vi "Set Pump Power.vi"(7 "timeout":i32=1000, 8 "error in":errorcluster, 9 "Power %":dbl=0.15 min=0.15 max=100.0 step=5.0 format="%#_2f", 11 "CAN Session In":T1) -> (0 "error out":errorcluster, 3 "CAN Session Out":T1)   [LabVIEW 2016]
uses:
  Program Files (x86)/National Instruments/LabVIEW 2016/examples/robotics/EPOS2 CANOpen Driver/Low Level VIs/Typedefs/CAN Refnum.ctl
  Program Files (x86)/National Instruments/LabVIEW 2016/examples/robotics/EPOS2 CANOpen Driver/Low Level VIs/Typedefs/CAN Session Pointer.ctl
  Program Files (x86)/National Instruments/LabVIEW 2016/examples/robotics/EPOS2 CANOpen Driver/Low Level VIs/Typedefs/CAN Communication References.ctl
  Program Files (x86)/National Instruments/LabVIEW 2016/examples/robotics/EPOS2 CANOpen Driver/Low Level VIs/Typedefs/kill process notifier array.ctl
  Program Files (x86)/National Instruments/LabVIEW 2016/examples/robotics/EPOS2 CANOpen Driver/Low Level VIs/Typedefs/Write Queue.ctl
  Program Files (x86)/National Instruments/LabVIEW 2016/examples/robotics/EPOS2 CANOpen Driver/Low Level VIs/Typedefs/FPGA CAN Frame Cluster.ctl
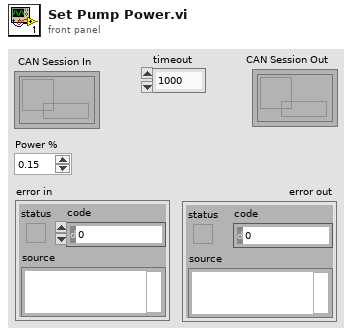
[diagram p1: front panel]
types:
  T1 = typedef "CAN Refnum.ctl" = refnum<k1>
  T2 = typedef "FPGA CAN Frame Cluster.ctl" = cluster{"Timestamp":u64, "Identifier":u32, "Type":u8, "InfoA":u8, "InfoB":u8, "DataLength":u8, "Data":u8[]}
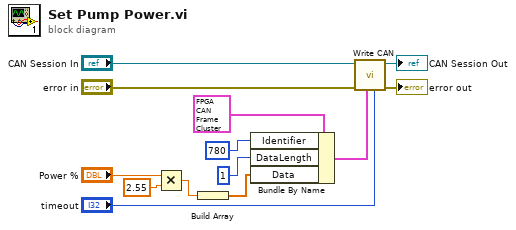
[diagram p0: block diagram]
diagram:
  n1 = Multiply(x="Power %", y=2.55) -> (x*y=w2:dbl)
  n2 = Build Array(w2) -> (w10:dbl[])
  n3 = Bundle By Name(cluster=T2 {"Timestamp"=0, "Identifier"=0, "Type"=0, "InfoA"=0, "InfoB"=0, "DataLength"=0, "Data"=[0, 0, 0, 0, 0, 0, 0, 0]} ("CAN Frame"), "Identifier"=u32 780, "DataLength"=u8 1, "Data"=w10) -> (w9:T2)
  n4 = call "Write CAN.vi"("timeout"="timeout", "CAN Frame"=w9, "error in"="error in", "CAN Session In"="CAN Session In") -> ("error out"=→"error out":errorcluster, "CAN Session Out"=→"CAN Session Out":T1)  [unwired: 6 in]
